vi "Open-PowerMeter.vi"() -> (0 "error out":errorcluster, 3 "VISA Refnum out":refnum<visa-resource-name>)   [LabVIEW 2021]
doc: "Open Power Meter\n\nAndré Romero - 2020\nandretec@ifsc.usp.br"
uses:
  Global variables.vi
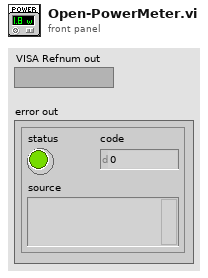
[diagram p1: front panel]
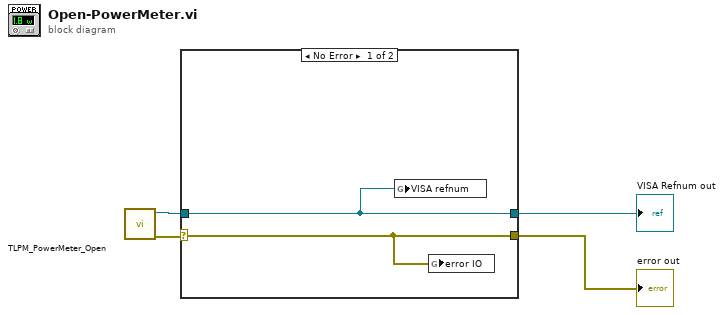
[diagram p0: block diagram]
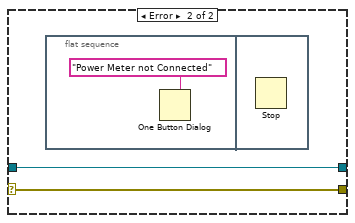
[diagram p2: hidden frame]
diagram:
  n1 = call "TLPM_PowerMeter_Open.vi"() -> ("error out"=w1:errorcluster, "instrument handle out"=w2:refnum<visa-resource-name>)  [unwired: 10 in]
  n2 = case shown="No Error" w1 {
    selector: w1 -> [w5 w8]
    tunnel: w2 -> [w6 w7]
    tunnel: [w6 w7] -> w3
    tunnel: [w5 w8] -> w4
    frame No Error {
      n3 = global write "Global variables.vi" "VISA refnum"(w6) -> ()
      n4 = global write "Global variables.vi" "error IO"(w5) -> ()
    }
    frame Error {
      n5 = flat-sequence {
        frame #0 {
          n6 = One Button Dialog(message="Power Meter not Connected") -> ()  [unwired: 1 in, 1 out]
        }
        frame #1 {
          n7 = Stop() -> ()  [unwired: 1 in]
        }
      }
    }
  }
  "error out" <- w4
  "VISA Refnum out" <- w3
